vi "Emballage_BDD_GVF_ImprimanteParDefaut.vi"(8 "Error in":errorcluster caption="Error in (no error)", 11 "SetGet":T1=enum."get") -> (0 "Error out":errorcluster, 2 "Imprimante Par defaut":string)   [LabVIEW 2020]
uses:
  Modules/FS/60_FS_Controles/60_FS_SetGet.ctl
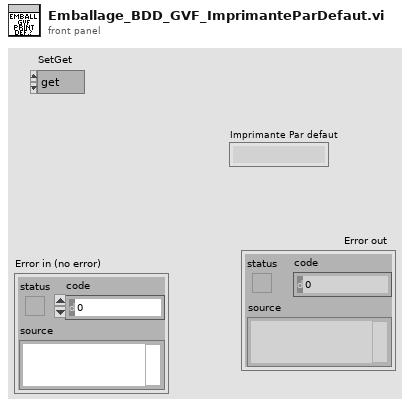
[diagram p1: front panel]
types:
  T1 = typedef "60_FS_SetGet.ctl" = enum16{"set", "get"}
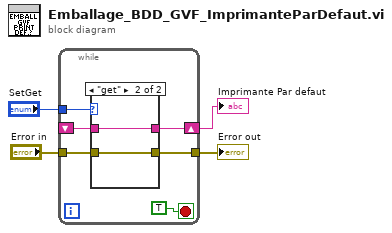
[diagram p0: block diagram]
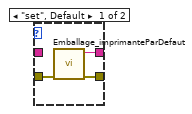
[diagram p2: hidden frame]
diagram:
  n1 = while {
    tunnel: "SetGet" -> [w9]
    shift-right: [w8] -> w3
    shift-left: _ -> [w7]
    tunnel: "Error in" -> [w6]
    tunnel: [w5] -> w1
    stop <- TRUE stop-if-true
    n2 = case shown="\"get\"" w9 {
      tunnel: [w13 w15] -> w8
      tunnel: w7 -> [_ w15]
      tunnel: w6 -> [w12 w14]
      tunnel: [w11 w14] -> w5
      frame "set", Default {
        n3 = call "Emballage_imprimanteParDefaut.vi"("Error in"=w12) -> ("Error out"=w11:errorcluster, "sous-chaîne suivante"=w13:string)  [unwired: 9 in]
      }
      frame "get" {
      }
    }
  }
  "Error out" <- w1
  "Imprimante Par defaut" <- w3
